vi "Gujar_Excersise1_121416.vi"   [LabVIEW 2014, in "Robo_Project.lvrbt"]
uses:
  Robo_Project/Robo_Project.lvrbt
  <vilib>/NXT/Block Support/NXT_OutputPort.ctl
  <vilib>/NXT/NXTIO Xnodes/NXTIONodeSubVIs/NXTMoveMotors.vi
  <vilib>/NXT/Dual Mode Library/Waits/Wait_Num.vi
  <vilib>/NXT/Subs/LVHSConnector.ctl
  <vilib>/NXT/NXTIO Xnodes/AddressXNode/NXTIOAddress.xnode
  <vilib>/NXT/NXTIO Xnodes/NXTIOXNode/NXTIO.xnode
  <vilib>/NXT/LegoClasses/BrickReference/BrickReference.lvclass
types:
  T1 = typedef "NXT_OutputPort.ctl" = u8
  T2 = typedef "LVHSConnector.ctl" = refnum<class "BrickReference.lvclass">
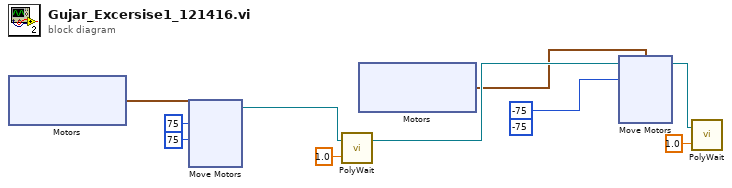
[diagram p0: block diagram]
diagram:
  (unwired) i8 -75 ("Power/Speed 2")
  n1 = xnode "Motors"() -> ("Motor"=w10:cluster{"Port":T1, "Port":T1})
  n2 = xnode "Move Motors"("Power/Speed 2"=i8 75, "Power/Speed 1"=i8 75, "Motors"=w10) -> ("NXT/EV3"=w6:T2)  [unwired: 1 in]
  n3 = call-poly <vilib>:"PolyWait.vi"("Time (1 sec)"=sgl 1.0, "NXT/EV3"=w6) -> ("NXT/EV3"=w2:T2)  [unwired: 2 in]
  n4 = xnode "Motors"() -> ("Motor"=w1:cluster{"Port":T1, "Port":T1})
  n5 = xnode "Move Motors"("Power/Speed 1"=i8 -75, "Motors"=w1, "NXT/EV3"=w2) -> ("NXT/EV3"=w3:T2)  [unwired: 1 in]
  n6 = call-poly <vilib>:"PolyWait.vi"("Time (1 sec)"=sgl 1.0, "NXT/EV3"=w3) -> ()  [unwired: 2 in, 1 out]
